vi "Part 2.vi"(11 "Input":string) -> (3 "Output":i64)   [LabVIEW 2021]
uses:
  7e16f333-fc4f-474c-b91f-87332ccbee1b.vi
  <userlib>/_OpenG.lib/string/string.llb/Convert EOLs (String)__ogtk.vi
  <vilib>/Comparison/Less/Less Functor/Less Functor.lvclass
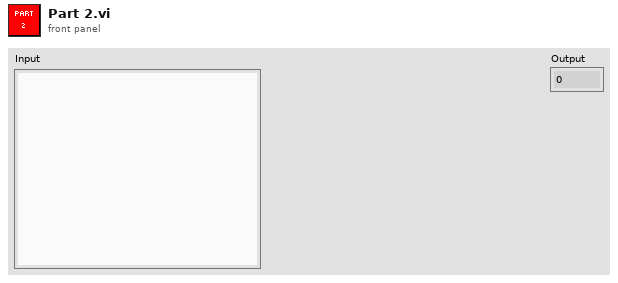
[diagram p1: front panel]
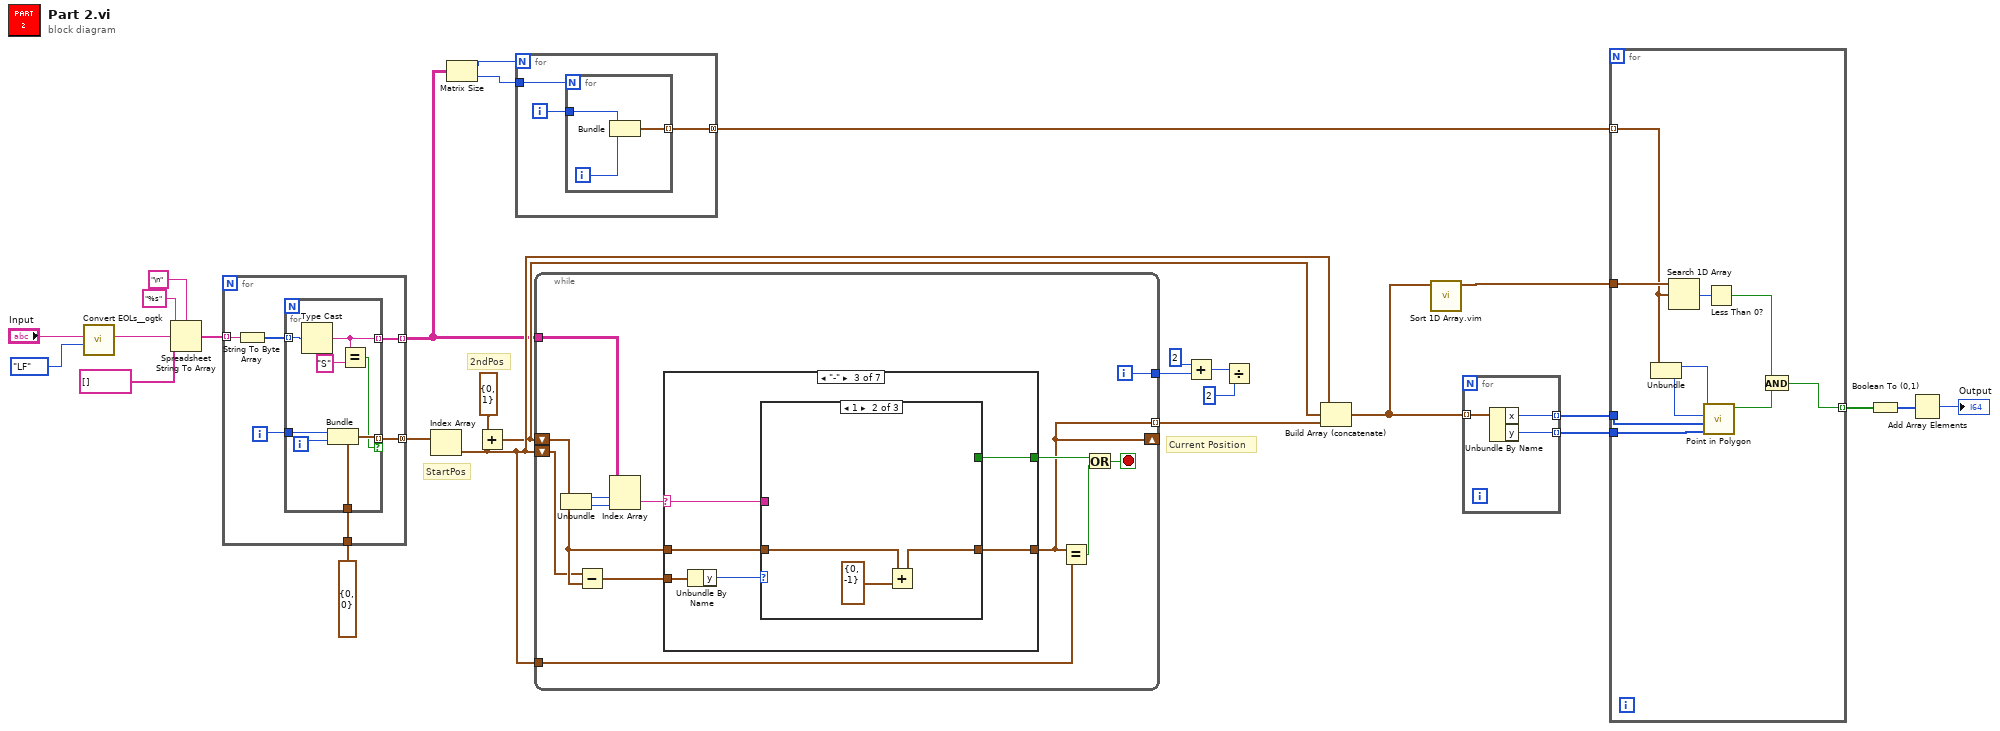
[diagram p0: block diagram]
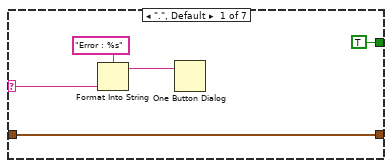
[diagram p2: hidden frame]
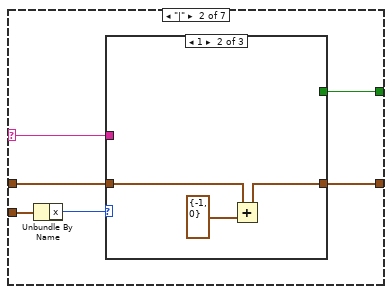
[diagram p3: hidden frame]
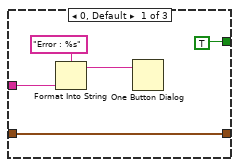
[diagram p4: hidden frame]
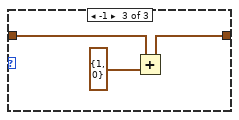
[diagram p5: hidden frame]
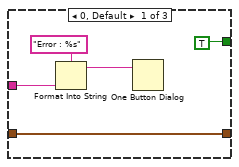
[diagram p6: hidden frame]
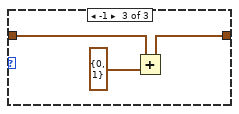
[diagram p7: hidden frame]
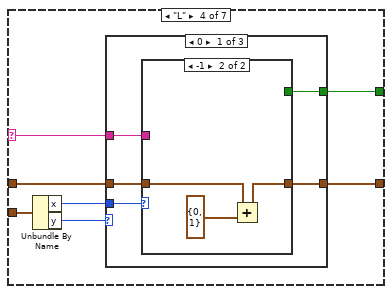
[diagram p8: hidden frame]
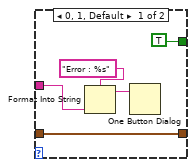
[diagram p9: hidden frame]
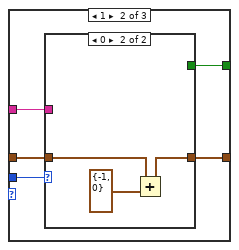
[diagram p10: hidden frame]
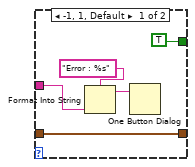
[diagram p11: hidden frame]
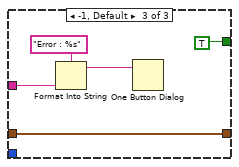
[diagram p12: hidden frame]
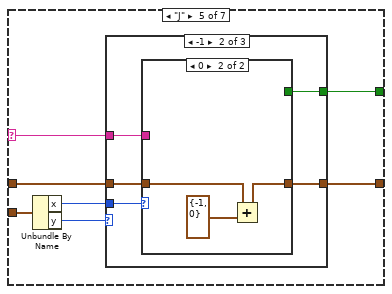
[diagram p13: hidden frame]
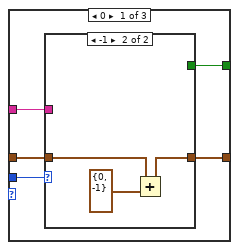
[diagram p14: hidden frame]
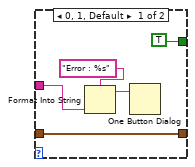
[diagram p15: hidden frame]
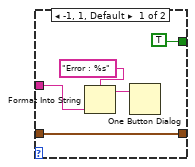
[diagram p16: hidden frame]
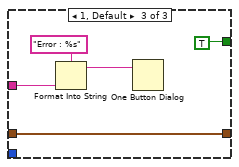
[diagram p17: hidden frame]
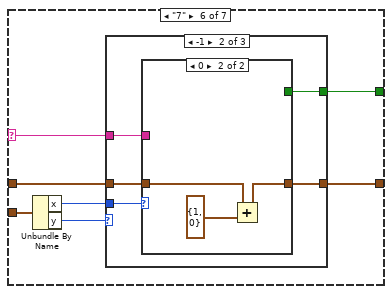
[diagram p18: hidden frame]
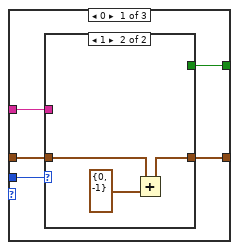
[diagram p19: hidden frame]
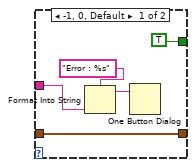
[diagram p20: hidden frame]
diagram:
  # "2ndPos"
  # "StartPos"
  # "Current Position"
  n1 = call-poly <userlib>:"Convert EOLs__ogtk.vi"("Convert to:"=enum16{"CR", "LF", "CRLF"}."LF", "String in"="Input") -> ("String out"=w24:string)  [unwired: 9 in]
  n2 = Spreadsheet String To Array(delimiter (Tab)="\n", format string="%s", spreadsheet string=w24, array type (2D Dbl)=string[] []) -> (array=w22:string[])
  n3 = for {
    tunnel: w22 -> [w34] mode=indexing
    tunnel: [w32] -> w11 mode=indexing
    tunnel: [w30] -> w21 mode=concatenating
    tunnel: cluster{"x":i32, "y":i32} {"x"=0, "y"=0} ("cluster") -> [w29]
    i -> [w31]
    n4 = String To Byte Array(string=w34) -> (unsigned byte array=w33:u8[])
    n5 = for {
      tunnel: w33 -> [w42] mode=indexing
      tunnel: [w41] -> w32 mode=indexing
      tunnel: w31 -> [w38]
      tunnel: [w37] -> w30 mode=indexing if=w36
      tunnel: w29 -> [w35]
      i -> [w39]
      n6 = Type Cast(x=w42) -> (*(type *) &x=w41:string)  [unwired: 1 in]
      n7 = Bundle(cluster=w35, "x"=w38, "y"=w39) -> (w37:cluster{"x":i32, "y":i32})
      n8 = Equal?(x=w41, y="S") -> (x = y?=w36:bool)
    }
  }
  n9 = Index Array(array=w21) -> (element=w14:cluster{"x":i32, "y":i32})  [unwired: 1 in]
  n10 = Matrix Size(0:w11) -> (1:w10:i32, 2:w5:i32)
  n11 = Add(x=cluster{i32, i32} {0, 1} ("y"), y=w14) -> (x+y=w13:cluster{i32, i32})
  n12 = for {
    N: w10 -> [_]
    tunnel: w5 -> [w45]
    tunnel: [w43] -> w9 mode=concatenating
    i -> [w44]
    n13 = for {
      N: w45 -> [_]
      tunnel: w44 -> [w48]
      tunnel: [w46] -> w43 mode=indexing
      i -> [w47]
      n14 = Bundle(w48, w47) -> (w46:cluster{i32, i32})  [unwired: 1 in]
    }
  }
  n15 = while {
    shift-right: [w49] -> _
    shift-left: w13 -> [w55]
    shift-left: w14 -> [w54]
    tunnel: w14 -> [w61]
    tunnel: [w60] -> w20
    tunnel: w11 -> [w59]
    tunnel: [w49] -> w15 mode=indexing
    i -> [w60]
    stop <- w52 stop-if-true
    n16 = Unbundle(w55) -> ("x"=w58:i32, "y"=w57:i32)
    n17 = Subtract(x=w54, y=w55) -> (x-y=w53:cluster{"x":i32, "y":i32})
    n18 = Index Array(array=w59, index (row)=w58, index (col)=w57) -> (element=w56:string)
    n19 = case shown="\"-\"" w56 {
      selector: w56 -> [w64 w67 w85 w103 w141 w179 w217]
      tunnel: w55 -> [w66 w70 w88 w106 w144 w182 w220]
      tunnel: [w66 w69 w87 w105 w143 w181 w219] -> w49
      tunnel: w53 -> [_ w72 w89 w107 w145 w183 w221]
      tunnel: [TRUE w68 w86 w104 w142 w180 w218] -> w51
      frame ".", Default {
        n20 = Format Into String(format string="Error : %s" ("message"), w64) -> (resulting string=w63:string)  [unwired: 2 in, 1 out]
        n21 = One Button Dialog(message=w63) -> ()  [unwired: 1 in, 1 out]
      }
      frame "|" {
        n22 = Unbundle By Name(w72) -> ("x"=w71:i32)
        n23 = case shown="1" w71 {
          tunnel: w70 -> [w77 w80 w83]
          tunnel: [w77 w79 w82] -> w69
          tunnel: [TRUE _ _] -> w68
          tunnel: w67 -> [w74 _ _]
          frame 0, Default {
            n24 = Format Into String(format string="Error : %s" ("message"), w74) -> (resulting string=w75:string)  [unwired: 2 in, 1 out]
            n25 = One Button Dialog(message=w75) -> ()  [unwired: 1 in, 1 out]
          }
          frame 1 {
            n26 = Add(x=w80, y=cluster{i32, i32} {-1, 0}) -> (x+y=w79:cluster{i32, i32})
          }
          frame -1 {
            n27 = Add(x=w83, y=cluster{i32, i32} {1, 0}) -> (x+y=w82:cluster{i32, i32})
          }
        }
      }
      frame "-" {
        n28 = Unbundle By Name(w89) -> ("y"=w84:i32)
        n29 = case shown="1" w84 {
          tunnel: w88 -> [w94 w97 w100]
          tunnel: [w94 w96 w99] -> w87
          tunnel: [TRUE _ _] -> w86
          tunnel: w85 -> [w91 _ _]
          frame 0, Default {
            n30 = Format Into String(format string="Error : %s" ("message"), w91) -> (resulting string=w92:string)  [unwired: 2 in, 1 out]
            n31 = One Button Dialog(message=w92) -> ()  [unwired: 1 in, 1 out]
          }
          frame 1 {
            n32 = Add(x=w97, y=cluster{i32, i32} {0, -1}) -> (x+y=w96:cluster{i32, i32})
          }
          frame -1 {
            n33 = Add(x=w100, y=cluster{i32, i32} {0, 1}) -> (x+y=w99:cluster{i32, i32})
          }
        }
      }
      frame "L" {
        n34 = Unbundle By Name(w107) -> ("x"=w101:i32, "y"=w102:i32)
        n35 = case shown="0" w102 {
          tunnel: w106 -> [w112 w125 w138]
          tunnel: [w111 w124 w138] -> w105
          tunnel: [w109 w122 TRUE] -> w104
          tunnel: w103 -> [w108 w121 w135]
          tunnel: w101 -> [w110 w123 _]
          frame 0 {
            n36 = case shown="-1" w110 {
              tunnel: w112 -> [w117 w120]
              tunnel: [w117 w119] -> w111
              tunnel: [TRUE _] -> w109
              tunnel: w108 -> [w113 _]
              frame 0, 1, Default {
                n37 = Format Into String(format string="Error : %s" ("message"), w113) -> (resulting string=w115:string)  [unwired: 2 in, 1 out]
                n38 = One Button Dialog(message=w115) -> ()  [unwired: 1 in, 1 out]
              }
              frame -1 {
                n39 = Add(x=w120, y=cluster{i32, i32} {0, 1}) -> (x+y=w119:cluster{i32, i32})
              }
            }
          }
          frame 1 {
            n40 = case shown="0" w123 {
              tunnel: w125 -> [w130 w133]
              tunnel: [w130 w132] -> w124
              tunnel: [TRUE _] -> w122
              tunnel: w121 -> [w126 _]
              frame -1, 1, Default {
                n41 = Format Into String(format string="Error : %s" ("message"), w126) -> (resulting string=w128:string)  [unwired: 2 in, 1 out]
                n42 = One Button Dialog(message=w128) -> ()  [unwired: 1 in, 1 out]
              }
              frame 0 {
                n43 = Add(x=w133, y=cluster{i32, i32} {-1, 0}) -> (x+y=w132:cluster{i32, i32})
              }
            }
          }
          frame -1, Default {
            n44 = Format Into String(format string="Error : %s" ("message"), w135) -> (resulting string=w136:string)  [unwired: 2 in, 1 out]
            n45 = One Button Dialog(message=w136) -> ()  [unwired: 1 in, 1 out]
          }
        }
      }
      frame "J" {
        n46 = Unbundle By Name(w145) -> ("x"=w139:i32, "y"=w140:i32)
        n47 = case shown="-1" w140 {
          tunnel: w144 -> [w150 w163 w176]
          tunnel: [w149 w162 w176] -> w143
          tunnel: [w147 w160 TRUE] -> w142
          tunnel: w141 -> [w146 w159 w173]
          tunnel: w139 -> [w148 w161 _]
          frame 0 {
            n48 = case shown="-1" w148 {
              tunnel: w150 -> [w155 w158]
              tunnel: [w155 w157] -> w149
              tunnel: [TRUE _] -> w147
              tunnel: w146 -> [w151 _]
              frame 0, 1, Default {
                n49 = Format Into String(format string="Error : %s" ("message"), w151) -> (resulting string=w153:string)  [unwired: 2 in, 1 out]
                n50 = One Button Dialog(message=w153) -> ()  [unwired: 1 in, 1 out]
              }
              frame -1 {
                n51 = Add(x=w158, y=cluster{i32, i32} {0, -1}) -> (x+y=w157:cluster{i32, i32})
              }
            }
          }
          frame -1 {
            n52 = case shown="0" w161 {
              tunnel: w163 -> [w168 w171]
              tunnel: [w168 w170] -> w162
              tunnel: [TRUE _] -> w160
              tunnel: w159 -> [w164 _]
              frame -1, 1, Default {
                n53 = Format Into String(format string="Error : %s" ("message"), w164) -> (resulting string=w166:string)  [unwired: 2 in, 1 out]
                n54 = One Button Dialog(message=w166) -> ()  [unwired: 1 in, 1 out]
              }
              frame 0 {
                n55 = Add(x=w171, y=cluster{i32, i32} {-1, 0}) -> (x+y=w170:cluster{i32, i32})
              }
            }
          }
          frame 1, Default {
            n56 = Format Into String(format string="Error : %s" ("message"), w173) -> (resulting string=w174:string)  [unwired: 2 in, 1 out]
            n57 = One Button Dialog(message=w174) -> ()  [unwired: 1 in, 1 out]
          }
        }
      }
      frame "7" {
        n58 = Unbundle By Name(w183) -> ("x"=w177:i32, "y"=w178:i32)
        n59 = case shown="-1" w178 {
          tunnel: w182 -> [w188 w201 w214]
          tunnel: [w187 w200 w214] -> w181
          tunnel: [w185 w198 TRUE] -> w180
          tunnel: w179 -> [w184 w197 w211]
          tunnel: w177 -> [w186 w199 _]
          frame 0 {
            n60 = case shown="1" w186 {
              tunnel: w188 -> [w193 w196]
              tunnel: [w193 w195] -> w187
              tunnel: [TRUE _] -> w185
              tunnel: w184 -> [w189 _]
              frame -1, 0, Default {
                n61 = Format Into String(format string="Error : %s" ("message"), w189) -> (resulting string=w191:string)  [unwired: 2 in, 1 out]
                n62 = One Button Dialog(message=w191) -> ()  [unwired: 1 in, 1 out]
              }
              frame 1 {
                n63 = Add(x=w196, y=cluster{i32, i32} {0, -1}) -> (x+y=w195:cluster{i32, i32})
              }
            }
          }
          frame -1 {
            n64 = case shown="0" w199 {
              tunnel: w201 -> [w206 w209]
              tunnel: [w206 w208] -> w200
              tunnel: [TRUE _] -> w198
              tunnel: w197 -> [w202 _]
              frame -1, 1, Default {
                n65 = Format Into String(format string="Error : %s" ("message"), w202) -> (resulting string=w204:string)  [unwired: 2 in, 1 out]
                n66 = One Button Dialog(message=w204) -> ()  [unwired: 1 in, 1 out]
              }
              frame 0 {
                n67 = Add(x=w209, y=cluster{i32, i32} {1, 0}) -> (x+y=w208:cluster{i32, i32})
              }
            }
          }
          frame 1, Default {
            n68 = Format Into String(format string="Error : %s" ("message"), w211) -> (resulting string=w212:string)  [unwired: 2 in, 1 out]
            n69 = One Button Dialog(message=w212) -> ()  [unwired: 1 in, 1 out]
          }
        }
      }
      frame "F" {
        n70 = Unbundle By Name(w221) -> ("x"=w215:i32, "y"=w216:i32)
        n71 = case shown="1" w216 {
          tunnel: w220 -> [w226 w239 w252]
          tunnel: [w225 w238 w252] -> w219
          tunnel: [w223 w236 TRUE] -> w218
          tunnel: w217 -> [w222 w235 w249]
          tunnel: w215 -> [w224 w237 _]
          frame 0 {
            n72 = case shown="1" w224 {
              tunnel: w226 -> [w231 w234]
              tunnel: [w231 w233] -> w225
              tunnel: [TRUE _] -> w223
              tunnel: w222 -> [w227 _]
              frame -1, 0, Default {
                n73 = Format Into String(format string="Error : %s" ("message"), w227) -> (resulting string=w229:string)  [unwired: 2 in, 1 out]
                n74 = One Button Dialog(message=w229) -> ()  [unwired: 1 in, 1 out]
              }
              frame 1 {
                n75 = Add(x=w234, y=cluster{i32, i32} {0, 1}) -> (x+y=w233:cluster{i32, i32})
              }
            }
          }
          frame 1 {
            n76 = case shown="0" w237 {
              tunnel: w239 -> [w244 w247]
              tunnel: [w244 w246] -> w238
              tunnel: [TRUE _] -> w236
              tunnel: w235 -> [w240 _]
              frame -1, 1, Default {
                n77 = Format Into String(format string="Error : %s" ("message"), w240) -> (resulting string=w242:string)  [unwired: 2 in, 1 out]
                n78 = One Button Dialog(message=w242) -> ()  [unwired: 1 in, 1 out]
              }
              frame 0 {
                n79 = Add(x=w247, y=cluster{i32, i32} {1, 0}) -> (x+y=w246:cluster{i32, i32})
              }
            }
          }
          frame -1, Default {
            n80 = Format Into String(format string="Error : %s" ("message"), w249) -> (resulting string=w250:string)  [unwired: 2 in, 1 out]
            n81 = One Button Dialog(message=w250) -> ()  [unwired: 1 in, 1 out]
          }
        }
      }
    }
    n82 = Equal?(x=w49, y=w61) -> (x = y?=w50:bool)
    n83 = Or(x=w51, y=w50) -> (x .or. y?=w52:bool)
  }
  n84 = Add(x=2, y=w20) -> (x+y=w18:i32)
  n85 = Divide(x=w18, y=2) -> ()  [unwired: 1 out]
  n86 = Build Array (concatenate)(w14, w13, w15) -> (w1:cluster{"x":i32, "y":i32}[])
  n87 = call "Sort 1D Array.vim"("unsorted array"=w1) -> ("sorted array"=w2:cluster{"x":i32, "y":i32}[])  [unwired: 10 in]
  n88 = for {
    tunnel: w1 -> [w255] mode=indexing
    tunnel: [w254] -> w4 mode=indexing
    tunnel: [w253] -> w3 mode=indexing
    n89 = Unbundle By Name(w255) -> ("x"=w254:i32, "y"=w253:i32)
  }
  n90 = for {
    tunnel: w9 -> [w260] mode=indexing
    tunnel: [w258] -> w6 mode=indexing
    tunnel: w4 -> [w265]
    tunnel: w3 -> [w264]
    tunnel: w2 -> [w261]
    n91 = Unbundle(w260) -> (w262:i32, w263:i32)
    n92 = Search 1D Array(1D array=w261, element=w260) -> (index of element=w257:i32)  [unwired: 1 in]
    n93 = call "Point in Polygon.vi"("polyY"=w264, "polyX"=w265, "y"=w263, "x"=w262) -> ("Inside?"=w259:bool)  [unwired: 7 in]
    n94 = Less Than 0?(x=w257) -> (x < 0?=w256:bool)
    n95 = And(x=w256, y=w259) -> (x .and. y?=w258:bool)
  }
  n96 = Boolean To (0,1)(Boolean=w6) -> (0, 1=w8:i16[])
  n97 = Add Array Elements(numeric array=w8) -> (sum=→"Output":i16)
